vi "S2C_XML_ManageLimits.vi"(6 "TagValue":string, 7 "Field":string, 8 "Error In":errorcluster, 9 "TagName":string, 10 "Meas In":refnum<k20>, 11 "Doc In":refnum<k20>) -> (0 "Error Out":errorcluster, 2 "Meas Out":refnum<k20>, 3 "Doc Out":refnum<k20>)   [LabVIEW 2015]
uses:
  S2C_XML_Globals.vi
  <resource>/objmgr/DOMUserDefRef.rc
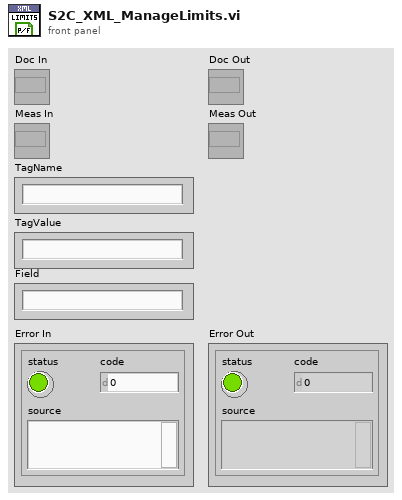
[diagram p1: front panel]
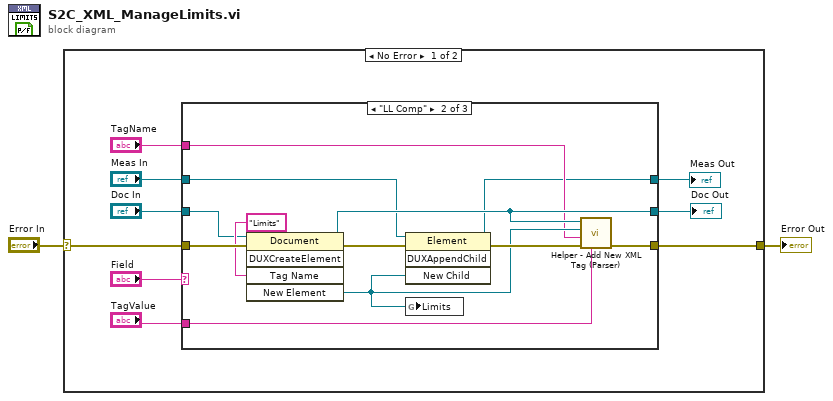
[diagram p0: block diagram]
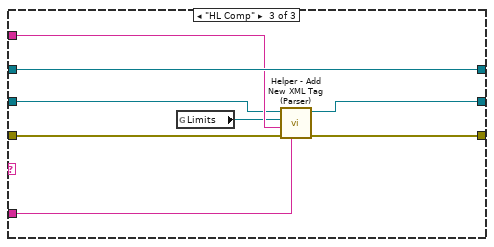
[diagram p3: hidden frame]
diagram:
  n1 = case shown="No Error" "Error In" {
    selector: "Error In" -> [w11 w35]
    tunnel: [w5 w35] -> w1
    frame No Error {
      n2 = case shown="\"LL Comp\"" "Field" {
        tunnel: w11 -> [w14 w26 w33]
        tunnel: [w14 w21 w29] -> w5
        tunnel: "Doc In" -> [w13 w20 w28]
        tunnel: [w13 w19 w27] -> w9
        tunnel: "Meas In" -> [w12 w18 w34]
        tunnel: [w12 w15 w34] -> w7
        tunnel: "TagValue" -> [_ w17 w32]
        tunnel: "TagName" -> [_ w16 w31]
        frame "Other", Default {
        }
        frame "LL Comp" {
          n3 = invoke class="Document" method="DUXCreateElement"(reference=w20, error in=w26, "Tag Name"="Limits") -> (reference out=w19:refnum<k20>, error out=w24:errorcluster, "New Element"=w22:refnum<k20>)  [unwired: 2 in, 2 out]
          n4 = invoke class="Element" method="DUXAppendChild"(reference=w18, error in=w24, "New Child"=w22) -> (reference out=w15:refnum<k20>, error out=w23:errorcluster)  [unwired: 1 in, 2 out]
          n5 = global write "S2C_XML_Globals.vi" "Limits"(w22) -> ()
          n6 = call "Helper - Add New XML Tag (Parser).vi"("Tag Data"=w17, "error in (no error)"=w23, "Tag Name"=w16, "Owning Element"=w22, "DOM document"=w19) -> ("error out"=w21:errorcluster)  [unwired: 4 in, 2 out]
        }
        frame "HL Comp" {
          n7 = global read "S2C_XML_Globals.vi" "Limits"() -> (w30:refnum<k20>)
          n8 = call "Helper - Add New XML Tag (Parser).vi"("Tag Data"=w32, "error in (no error)"=w33, "Tag Name"=w31, "Owning Element"=w30, "DOM document"=w28) -> ("error out"=w29:errorcluster, "dup DOM document"=w27:refnum<k20>)  [unwired: 4 in, 1 out]
        }
      }
      "Doc Out" <- w9
      "Meas Out" <- w7
    }
    frame Error {
    }
  }
  "Error Out" <- w1
